vi "Test Work Dispatcher Forward Message.vi"(8 "error in (no error)":errorcluster, 11 "Work Dispatcher Test in":refnum<class "Work Dispatcher Test.lvclass">=refnum) -> (0 "error out":errorcluster, 3 "Work Dispatcher Test out":refnum<class "Work Dispatcher Test.lvclass">)   [LabVIEW 2020, in "Work Dispatcher Test.lvclass"]
uses:
  Work Dispatcher Test.lvclass
  <vilib>/Astemes/Triarc Framework/Process/Process.lvclass
  Processes/Work Dispatcher/Work Dispatcher.lvclass
  Test Doubles/Mock Job Handler/Mock Job Handler.lvclass
  <vilib>/Astemes/LUnit/Test Case.lvclass
  C:/Program Files (x86)/National Instruments/LabVIEW 2020/vi.lib/Astemes/Triarc Framework/Process/Process.lvclass
  C:/Program Files (x86)/National Instruments/LabVIEW 2020/vi.lib/Astemes/Triarc Framework/Base/Base.lvclass
  C:/Program Files (x86)/National Instruments/LabVIEW 2020/vi.lib/Astemes/Triarc Framework/Error Handler Interface/Error Handler Interface.lvclass
  C:/Program Files (x86)/National Instruments/LabVIEW 2020/vi.lib/Astemes/Triarc Framework/Logging/Logging.lvclass
  C:/git/astemes-triarc-examples/source/Coffee Shop/Processes/Work Dispatcher/Work Dispatcher.lvclass
  C:/git/astemes-triarc-examples/source/Coffee Shop/Processes/People/Process Job/Job Handler.lvclass
  C:/Program Files (x86)/National Instruments/LabVIEW 2020/vi.lib/Astemes/Triarc Framework/Helper Loop/Helper Loop.lvclass
  C:/Program Files (x86)/National Instruments/LabVIEW 2020/vi.lib/Astemes/LUnit/Test Case.lvclass
  C:/Program Files (x86)/National Instruments/LabVIEW 2020/vi.lib/Astemes/LUnit/LUnit Runnable.lvclass
  C:/git/astemes-triarc-examples/source/Coffee Shop/Tests/Test Doubles/Mock Job Handler/Mock Job Handler.lvclass
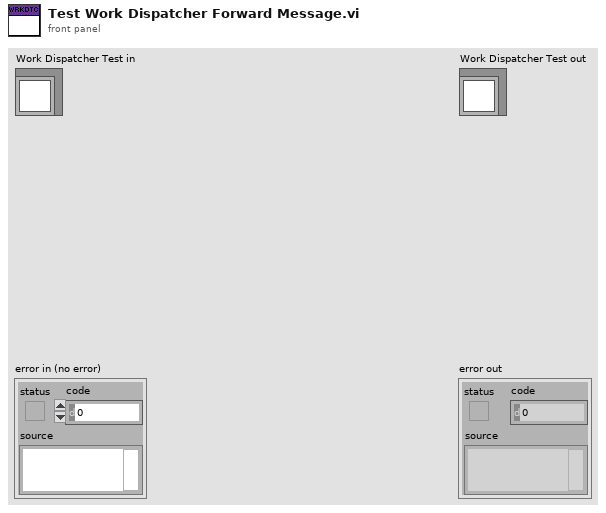
[diagram p1: front panel]
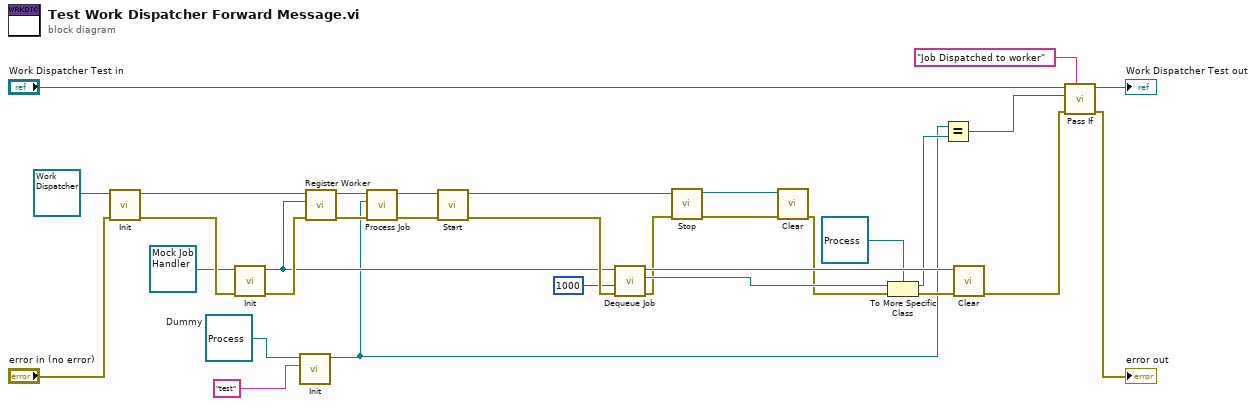
[diagram p0: block diagram]
diagram:
  w15 = refnum<class "Process.lvclass"> refnum  # Dummy
  n1 = call-dynamic "Init.vi"("error in (no error)"="error in (no error)", "Process In"=refnum<class "Work Dispatcher.lvclass"> refnum ("Work Dispatcher.lvclass")) -> ("error out"=w29:errorcluster, "Process Out"=w30:refnum<class "Work Dispatcher.lvclass">)  [unwired: 8 in]
  n2 = call-dynamic "Init.vi"("error in (no error)"=w29, "Mock Job Handler In"=refnum<class "Mock Job Handler.lvclass"> refnum ("Mock Worker In")) -> ("error out"=w22:errorcluster, "Mock Job Handler Out"=w16:refnum<class "Mock Job Handler.lvclass">)  [unwired: 8 in]
  n3 = call-dynamic "Init.vi"("Name"="test", "Process In"=w15) -> ("Process Out"=w3:refnum<class "Process.lvclass">)  [unwired: 8 in, 1 out]
  n4 = call-dynamic "Register Worker.vi"("error in (no error)"=w22, "Worker"=w16, "Work Dispatcher In"=w30) -> ("error out"=w20:errorcluster, "Work Dispatcher Out"=w21:refnum<class "Work Dispatcher.lvclass">)  [unwired: 7 in]
  n5 = call-dynamic "Process Job.vi"("error in (no error)"=w20, "Task"=w3, "Work Dispatcher In"=w21) -> ("error out"=w18:errorcluster, "Work Dispatcher Out"=w19:refnum<class "Work Dispatcher.lvclass">)  [unwired: 7 in]
  n6 = call <vilib>:"Start.vi"("error in (no error)"=w18, "Process In"=w19) -> ("error out"=w23:errorcluster, "Process Out"=w28:refnum<class "Work Dispatcher.lvclass">)  [unwired: 7 in, 1 out]
  n7 = call "Dequeue Job.vi"("error in (no error)"=w23, "timeout in ms (-1)"=1000, "Mock Job Handler In"=w16) -> ("error out"=w7:errorcluster, "element"=w14:refnum<class>, "Mock Job Handler Out"=w24:refnum<class "Mock Job Handler.lvclass">)  [unwired: 5 in, 1 out]
  n8 = call <vilib>:"Stop.vi"("error in (no error)"=w7, "Process In"=w28) -> ("error out"=w26:errorcluster, "Process Out"=w27:refnum<class "Work Dispatcher.lvclass">)  [unwired: 7 in, 1 out]
  n9 = call-dynamic "Clear.vi"("error in (no error)"=w26, "Process In"=w27) -> ("error out"=w5:errorcluster)  [unwired: 9 in]
  n10 = To More Specific Class(target class=refnum<class "Process.lvclass"> refnum, reference=w14, error in=w5) -> (specific class reference=w6:refnum<class "Process.lvclass">, error out=w4:errorcluster)
  n11 = Equal?(x=w3, y=w6) -> (x = y?=w11:bool)
  n12 = call-dynamic "Clear.vi"("error in (no error)"=w4, "Mock Job Handler In"=w24) -> ("error out"=w10:errorcluster)  [unwired: 9 in]
  n13 = call <vilib>:"Pass If.vi"("Description"="Job Dispatched to worker", "error in (no error)"=w10, "Pass?"=w11, "LUnit Test Case In"="Work Dispatcher Test in") -> ("error out"=→"error out":errorcluster, "LUnit Test Case Out"=→"Work Dispatcher Test out":refnum<class "Test Case.lvclass">)  [unwired: 6 in]
